vi "Mysql data reader 1D integer.vi"(8 "error in (no error)":errorcluster, 11 ".NET Refnum in":refnum<k24>) -> (0 "error out":errorcluster, 3 "Array":i32[](array[numeric]))   [LabVIEW 2020, in "mysql.lvlib" / "mysql.lvclass"]
uses:
  mysql.lvclass
  MySql.Data
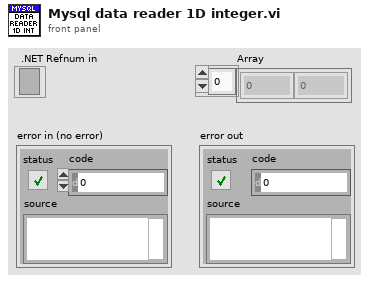
[diagram p1: front panel]
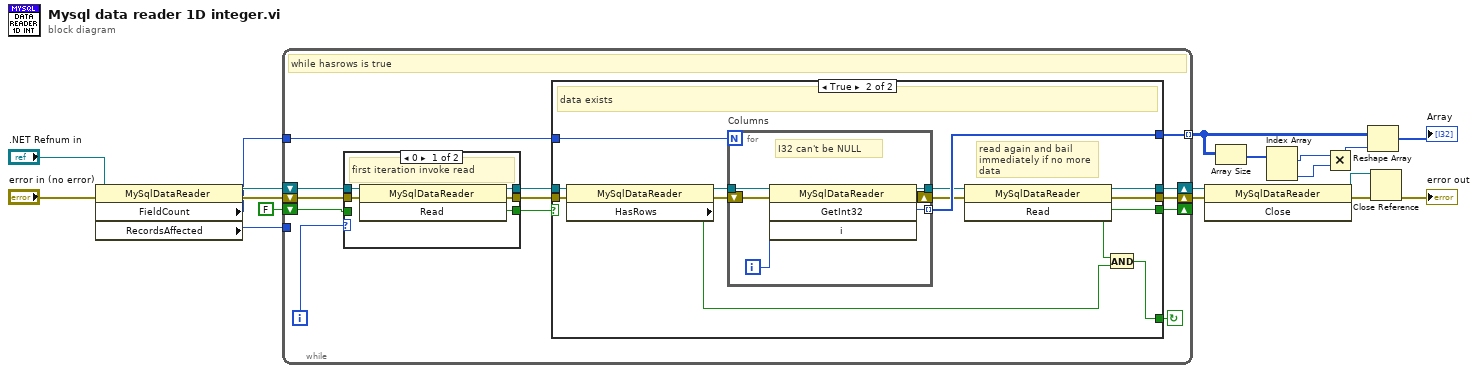
[diagram p0: block diagram]
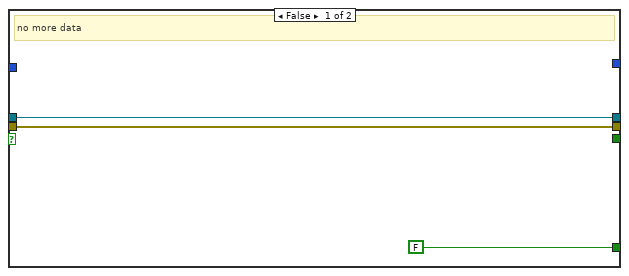
[diagram p3: hidden frame]
diagram:
  n1 = property class="MySqlDataReader"(reference=".NET Refnum in", error in="error in (no error)") -> (reference out=w13:refnum<k24>, error out=w12:errorcluster, "FieldCount"=w10:i32, "RecordsAffected"=w18:i32)
  n2 = while {
    tunnel: w10 -> [w31]
    tunnel: [w30] -> w3 mode=indexing
    shift-right: [w28] -> w15
    shift-left: w12 -> [w26]
    shift-right: [w29] -> w14
    shift-left: w13 -> [w25]
    tunnel: w18 -> [_]
    shift-right: [w20] -> _
    shift-left: FALSE ("Read") -> [w19]
    i -> [w24]
    stop <- w27 continue-if-true
    # "while hasrows is true"
    n3 = case shown="0" w24 {
      tunnel: w26 -> [w36 w38]
      tunnel: [w35 w38] -> w23
      tunnel: w25 -> [w34 w39]
      tunnel: [w33 w39] -> w22
      tunnel: [w32 w37] -> w21
      tunnel: w19 -> [_ w37]
      frame 0 {
        # "first iteration invoke read"
        n4 = invoke class="MySqlDataReader" method="Read"(reference=w34, error in=w36) -> (reference out=w33:refnum<k24>, error out=w35:errorcluster, "Read"=w32:bool)  [unwired: 1 in]
      }
      frame 1.., Default {
        # "read after for other iterations"
      }
    }
    n5 = case shown="True" w21 {
      tunnel: w31 -> [_ w55]
      tunnel: [_ w54] -> w30
      tunnel: w23 -> [w41 w53]
      tunnel: w22 -> [w42 w52]
      tunnel: [w42 w49] -> w29
      tunnel: [w41 w46] -> w28
      tunnel: [FALSE ("HasRows") w43] -> w27
      tunnel: [_ w45] -> w20
      frame False {
        # "no more data"
      }
      frame True {
        # "read again and bail immediately if no more data"
        # "data exists"
        n6 = property class="MySqlDataReader"(reference=w52, error in=w53) -> (reference out=w51:refnum<k24>, error out=w50:errorcluster, "HasRows"=w44:bool)
        n7 = for "Columns" {
          N: w55 -> [_]
          tunnel: w51 -> [w56]
          shift-right: [w61] -> w47
          shift-left: w50 -> [w57]
          tunnel: [w60] -> w54 mode=indexing
          tunnel: [w59] -> w48
          i -> [w58]
          # "I32 can't be NULL"
          n8 = invoke class="MySqlDataReader" method="GetInt32"(reference=w56, error in=w57, "i"=w58) -> (reference out=w59:refnum<k24>, error out=w61:errorcluster, "GetInt32"=w60:i32)  [unwired: 1 in, 1 out]
        }
        n9 = invoke class="MySqlDataReader" method="Read"(reference=w48, error in=w47) -> (reference out=w49:refnum<k24>, error out=w46:errorcluster, "Read"=w45:bool)  [unwired: 1 in]
        n10 = And(x=w45, y=w44) -> (x .and. y?=w43:bool)
      }
    }
  }
  n11 = invoke class="MySqlDataReader" method="Close"(reference=w14, error in=w15) -> (reference out=w17:refnum<k24>, error out=w16:errorcluster)  [unwired: 1 in, 1 out]
  n12 = Array Size(array=w3) -> (size(s)=w6:i32[])
  n13 = Index Array(array=w6) -> (element #1=w5:i32, element #2=w4:i32)  [unwired: 2 in]
  n14 = Multiply(x=w5, y=w4) -> (x*y=w2:i32)
  n15 = Reshape Array(w3, w2) -> (→"Array":i32[])
  n16 = Close Reference(reference=w17, error in (no error)=w16) -> (error out=→"error out":errorcluster)
